vi "SetBuildVersion.vi"(6 "Version (delimited)":string[](array[string]), 8 "error in (no error)":errorcluster, 9 "Target Name":string, 10 "Name of build specification":string, 11 "Path to project":path) -> (0 "error out":errorcluster, 1 "Set Version":T1)   [LabVIEW 2020]
doc: "Sets the version of the build specification based on the Version input or if no input is given, it gets the current version of the build specification and sets it."
uses:
  <vilib>/AppBuilder/AB_API_Simple/Build Specification Version.ctl
  <vilib>/AppBuilder/AB_API_Simple/NI_App_Builder_API.lvlib
  <vilib>/AppBuilder/AB_API_Simple/Set Build Specification Version (path).vi
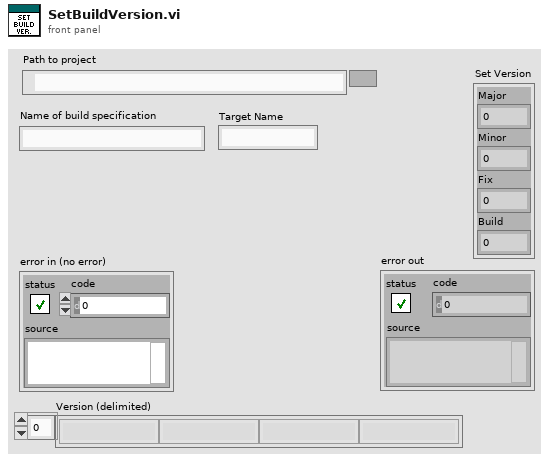
[diagram p1: front panel]
types:
  T1 = typedef "NI_App_Builder_API.lvlib/Build Specification Version.ctl" = cluster{"Major":u16, "Minor":u16, "Fix":u16, "Build":u16}
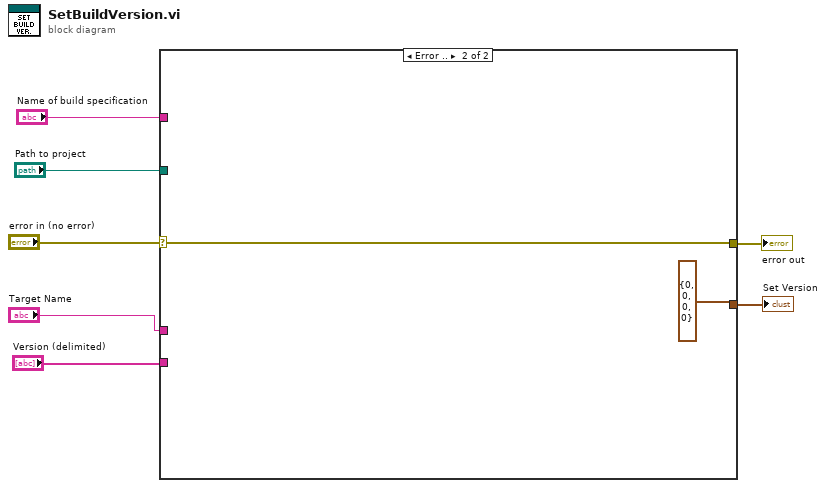
[diagram p0: block diagram]
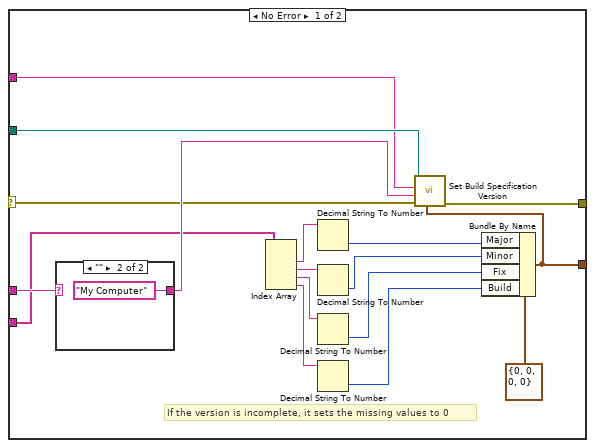
[diagram p2: hidden frame]
diagram:
  n1 = case shown="Error .." "error in (no error)" {
    selector: "error in (no error)" -> [w8 w28]
    tunnel: [w23 T1 {"Major"=0, "Minor"=0, "Fix"=0, "Build"=0} ("Build Specification Version")] -> w7
    tunnel: [w22 w28] -> w6
    tunnel: "Path to project" -> [w16 _]
    tunnel: "Target Name" -> [w11 _]
    tunnel: "Name of build specification" -> [w10 _]
    tunnel: "Version (delimited)" -> [w9 _]
    frame No Error {
      # "If the version is incomplete, it sets the missing values to 0"
      n2 = case shown="\"\"" w11 {
        selector: w11 -> [w25 _]
        tunnel: [w25 "My Computer"] -> w17
        frame Default {
        }
        frame "" {
        }
      }
      n3 = Index Array(array=w9) -> (element #1=w15:string, element #2=w12:string, element #3=w13:string, element #4=w14:string)  [unwired: 4 in]
      n4 = Decimal String To Number(string=w15) -> (number=w18:i32)  [unwired: 2 in, 1 out]
      n5 = Decimal String To Number(string=w12) -> (number=w19:i32)  [unwired: 2 in, 1 out]
      n6 = Decimal String To Number(string=w13) -> (number=w20:i32)  [unwired: 2 in, 1 out]
      n7 = Decimal String To Number(string=w14) -> (number=w21:i32)  [unwired: 2 in, 1 out]
      n8 = Bundle By Name(cluster=T1 {"Major"=0, "Minor"=0, "Fix"=0, "Build"=0} ("Build Specification Version"), "Major"=w18, "Minor"=w19, "Fix"=w20, "Build"=w21) -> (w23:T1)
      n9 = call-poly <vilib>:"Set Build Specification Version.vi"("Build Specification Version"=w23, "error in (no error)"=w8, "Name of target (My Computer)"=w17, "Name of build specification"=w10, "Path to project"=w16) -> ("error out"=w22:errorcluster)  [unwired: 6 in]
    }
    frame Error {
    }
  }
  "Set Version" <- w7
  "error out" <- w6
